vi "Create Measurement Plugin subVIs.vi"(11 "error in (no error)":errorcluster) -> (15 "error out":errorcluster)   [LabVIEW 2021, in "Converter.lvlib"]
uses:
  Converter.lvlib
  Path Functions/Path Functions.lvlib
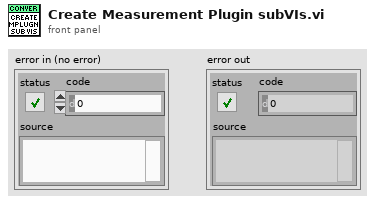
[diagram p1: front panel]
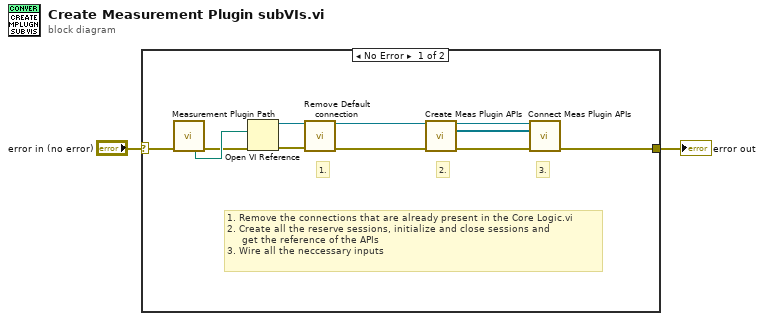
[diagram p0: block diagram]
diagram:
  n1 = case shown="No Error" "error in (no error)" {
    selector: "error in (no error)" -> [w10 w14]
    tunnel: [w5 w14] -> w2
    frame No Error {
      # "1. Remove the connections that are already present in the Core Logic.vi\n2. Create all the reserve sessions, initialize and close sessions and\n     get the reference of the APIs\n3. Wire all the neccessary inputs"
      # "3."
      # "2."
      # "1."
      n2 = call "Measurement Plugin Path.vi"("error in (no error)"=w10) -> ("Logic VI Path"=w11:path, "error out"=w9:errorcluster)  [unwired: 2 in, 11 out]
      n3 = Open VI Reference(vi path=w11, error in (no error)=w9) -> (vi reference=w13:refnum<vi>, error out=w12:errorcluster)  [unwired: 4 in]
      n4 = call "Remove Default connection.vi"("vi reference"=w13, "error in (no error)"=w12) -> ("vi reference out"=w7:refnum<vi>, "error out"=w8:errorcluster)  [unwired: 12 in]
      n5 = call "Create Meas Plugin APIs.vi"("Logic VI Ref"=w7, "error in (no error)"=w8) -> ("Logic VI Out"=w4:refnum<vi>, "SubVI Refrences"=w3:refnum<vi>[], "error out"=w6:errorcluster)  [unwired: 11 in]
      n6 = call "Connect Meas Plugin APIs.vi"("Logic VI Ref"=w4, "SubVIs"=w3, "error in (no error)"=w6) -> ("error out"=w5:errorcluster)  [unwired: 12 in]
    }
    frame Error {
    }
  }
  "error out" <- w2
